vi "LVClass_HasoData Read HasoData - property.vi"(8 "error in (no error)":errorcluster, 11 "HasoData in":refnum<class "HasoData.lvclass">) -> (0 "error out":errorcluster, 2 "HasoData":i32, 3 "HasoData out":refnum<class "HasoData.lvclass">)   [LabVIEW 2020, in "HasoData.lvclass"]
uses:
  HasoData.lvclass
  HasoData.lvclass/HasoData.ctl
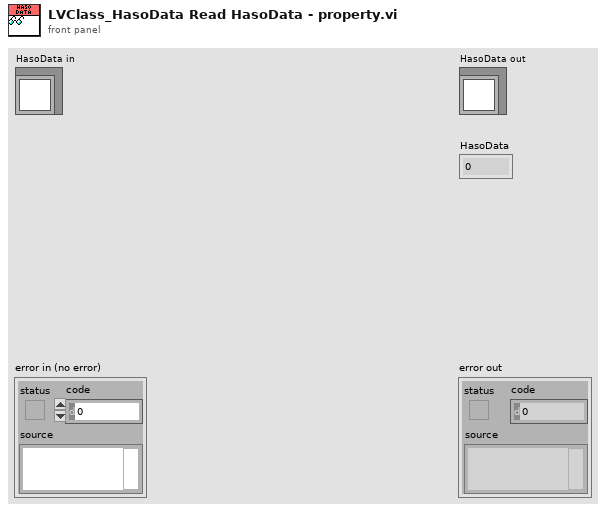
[diagram p1: front panel]
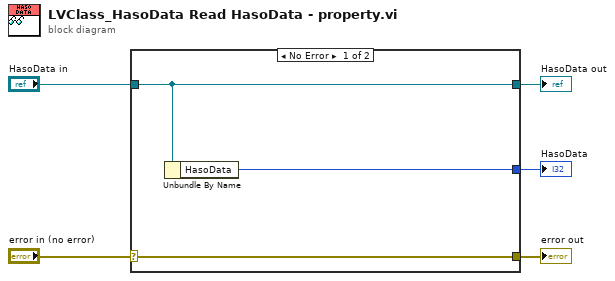
[diagram p0: block diagram]
diagram:
  n1 = case shown="No Error" "error in (no error)" {
    selector: "error in (no error)" -> [w8 w9]
    tunnel: [w8 w9] -> w4
    tunnel: [w7 w10] -> w2
    tunnel: "HasoData in" -> [w7 w10]
    tunnel: [w6 _] -> w1
    frame No Error {
      n2 = Unbundle By Name(w7) -> ("HasoData"=w6:i32)
    }
    frame Error {
    }
  }
  "error out" <- w4
  "HasoData out" <- w2
  "HasoData" <- w1
